vi "FindStartEndPointsRRTImproved.vi"(5 "Robot in":T1, 6 "enemy_robots":T1[](array[typedef]), 7 "ball":dbl[](array[numeric]), 8 "our_robots":T1[](array[typedef]), 9 "Goal":dbl[](array[numeric]), 10 "Initial State":dbl[](array[numeric]), 11 "Collision Points":dbl[][](array[numeric])) -> (2 "Start End Points RRT":dbl[][](array[numeric]))   [LabVIEW 2017]
uses:
  Core/AI Robot.ctl
  Intel/Functions Enum.ctl
  Intel/AttackerStates.ctl
  PathDests.ctl
  PathDest.ctl
  <vilib>/Analysis/_algsub.llb/Real Vector Norm.vi
  <vilib>/Analysis/NI_AALPro.lvlib
panel:
  in  "tamanho minimo":dbl=300.0 format="%#_13g"
  in  "threshold":dbl=50.0 format="%#_13g"
  out "Collision Points \nordenado":dbl[][](array[numeric])
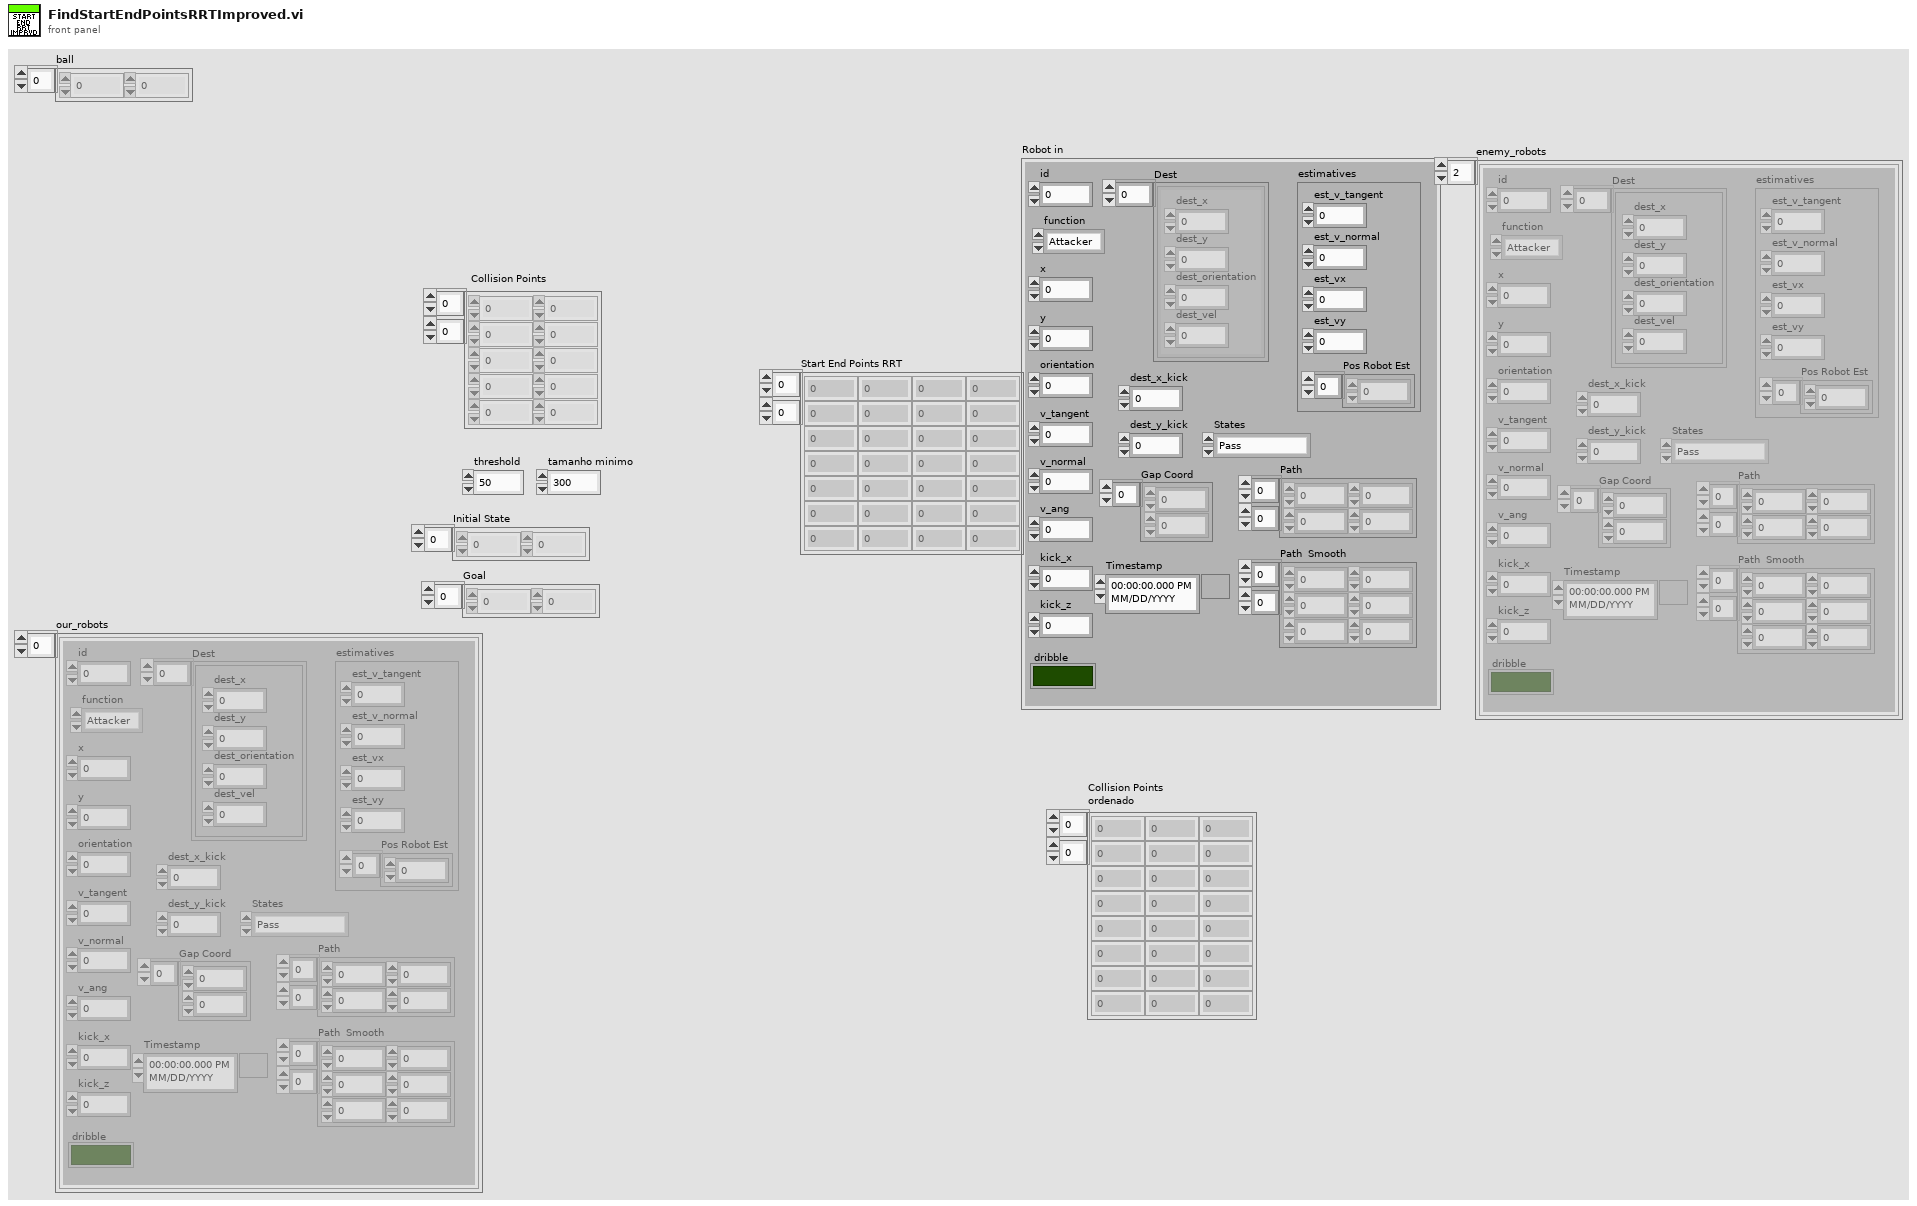
[diagram p1: front panel]
types:
  T1 = typedef "AI Robot.ctl" = cluster{"id":u32, "function":T2, "x":dbl, "y":dbl, "orientation":dbl, "v_tangent":dbl, "v_normal":dbl, "v_ang":dbl, "kick_x":dbl, "kick_z":dbl, "dribble":bool, "Timestamp":timestamp, "estimatives":cluster{"est_v_tangent":dbl, "est_v_normal":dbl, "est_vx":dbl, "est_vy":dbl, "Pos Robot Est":dbl[]}, "dest_x_kick":dbl, "dest_y_kick":dbl, "Gap Coord":dbl[], "States":T3, "Path ":dbl[][], "Path  Smooth":dbl[][], "Dest":T4}
  T2 = typedef "Functions Enum.ctl" = enum16{"Attacker", "Goalie", "Defender", "Striker", "Goto 0", "Dummy", "Kicker", "ZigZag 0", "ZigZag 1", "ZigZag 2", "ZigZag 3", "ZigZag 4", "ZigZag 5", "ZigZag 6", "ZigZag 7", "ZigZag 8", ""}
  T3 = typedef "AttackerStates.ctl" = enum16{"Pass", "GoToTangent", "BallGetting", "GoToKick", ""}
  T4 = typedef "PathDests.ctl" = T5[]
  T5 = typedef "PathDest.ctl" = cluster{"dest_x":dbl, "dest_y":dbl, "dest_orientation":dbl, "dest_vel":dbl}
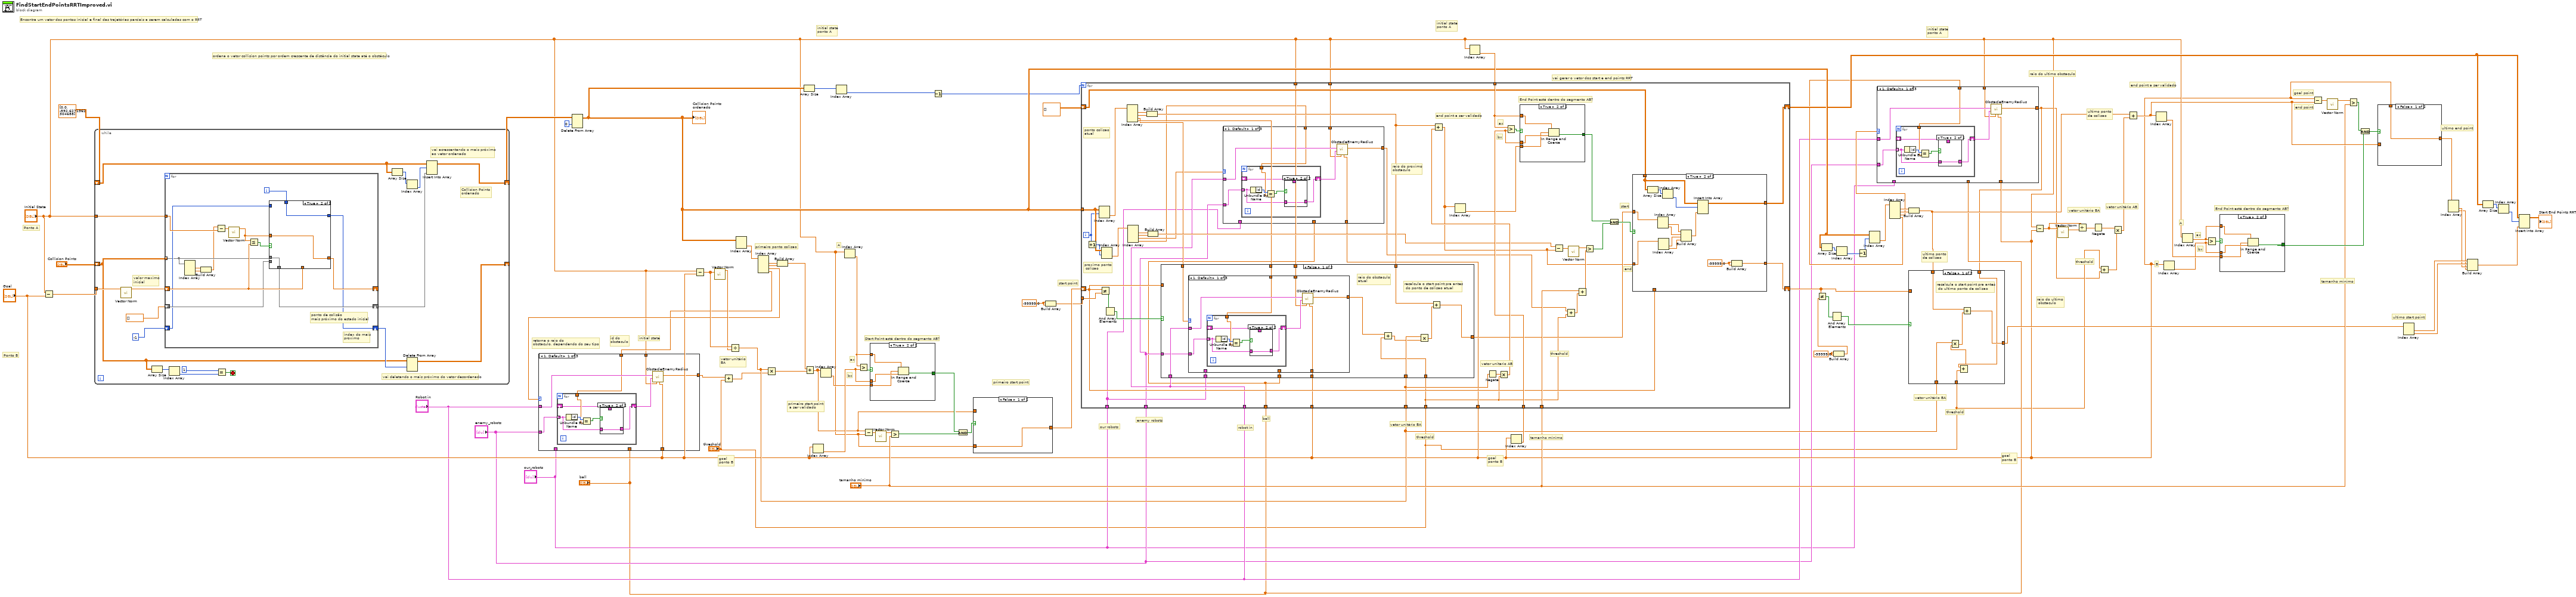
[diagram p0: block diagram]
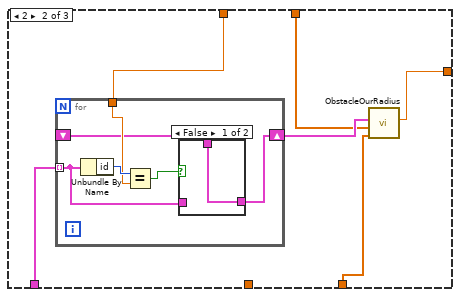
[diagram p3: hidden frame]
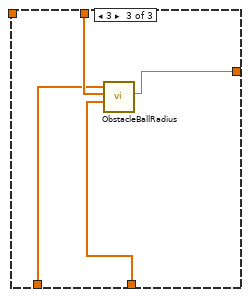
[diagram p5: hidden frame]
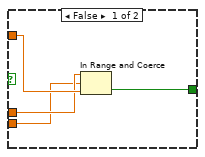
[diagram p6: hidden frame]
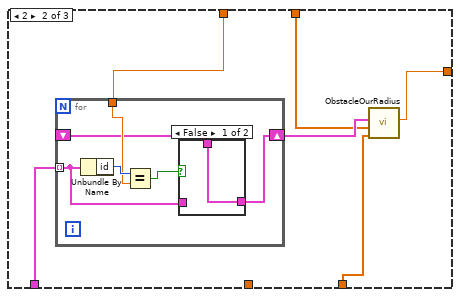
[diagram p10: hidden frame]
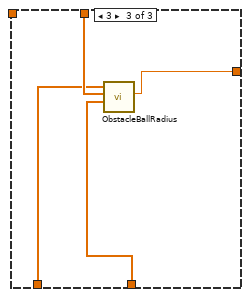
[diagram p12: hidden frame]
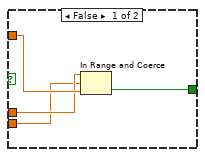
[diagram p14: hidden frame]
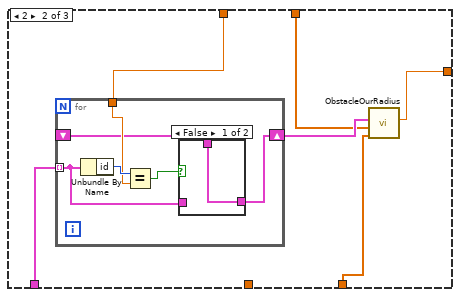
[diagram p16: hidden frame]
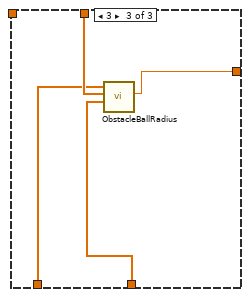
[diagram p18: hidden frame]
diagram:
  w46 = -99999.0 ("element")
  w51 = -99999.0 ("element")
  # "raio do ultimo\n obstaculo"
  # "raio do ultimo obstaculo"
  # "ball"
  # "robot in"
  # "enemy robots"
  # "our robots"
  # "initial state"
  # "id do\nobstaculo"
  # "retorna o raio do \nobstaculo, dependendo do seu tipo"
  # "vai gerar o vetor dos start e end points RRT"
  # "ultimo start point"
  # "ultimo end point"
  # "tamanho minimo"
  # "end point a ser validado"
  # "ultimo ponto\nde colisao"
  # "threshold"
  # "goal\nponto B"
  # "initial state\nponto A"
  # "ultimo ponto\nde colisao"
  # "threshold"
  # "vetor unitário BA"
  # "tamanho minimo"
  # "initial state\nponto A"
  # "goal\nponto B"
  # "threshold"
  # "vetor unitário BA"
  # "start point"
  # "primeiro start point"
  # "A"
  # "Start Point está dentro do segmento AB?"
  # "bx"
  # "ax"
  # "primeiro start point\n a ser validado"
  # "primeiro ponto colisao"
  # "vetor unitário\nBA"
  # "initial state\nponto A"
  # "goal\nponto B"
  # "ordena o vetor collision points por ordem crescente de distância do initial state até o obstáculo"
  # "Encontra um vetor dos pontos inicial e final das trajetórias parciais a serem calculadas com o RRT"
  # "end point"
  # "goal point"
  # "End Point está dentro do segmento AB?"
  # "bx"
  # "ax"
  # "B"
  # "A"
  # "vetor unitário AB"
  # "vetor unitário BA"
  # "Ponto B"
  # "Ponto A"
  n1 = Subtract(x="Initial State", y="Goal") -> (x-y=w87:dbl[])
  n2 = while {
    tunnel: w87 -> [w104]
    tunnel: "Initial State" -> [w101]
    shift-right: [w97] -> w68
    shift-left: dbl[][] [[0.0, -592.6271362304688]] ("Collision Points") -> [w99]
    shift-right: [w93] -> _
    shift-left: "Collision Points" -> [w92]
    stop <- w89 stop-if-true
    # "vai acrescentando o mais próximo\nao vetor ordenado"
    # "vai deletando o mais próximo do vetor desordenado"
    # "Collision Points \nordenado"
    # "valor maximo\ninicial"
    n3 = call-poly <vilib>:"Vector Norm.vi"("Input Vector"=w104) -> ("norm"=w103:dbl)  [unwired: 9 in, 1 out]
    n4 = Array Size(array=w92) -> (size(s)=w91:i32[])
    n5 = for {
      tunnel: w92 -> [w108] mode=indexing
      tunnel: w101 -> [w112]
      shift-right: [w116] -> _
      shift-left: w103 -> [w117]
      shift-right: [w115] -> w98
      shift-left: dbl[] [] ("Goal 2") -> [w114]
      shift-right: [w110] -> w94
      shift-left: -1 -> [w109]
      i -> [w111]
      # "index do mais\nproximo"
      # "ponto de colisão \nmais próximo do estado inicial"
      n6 = Index Array(array=w108) -> (element #1=w107:dbl, element #2=w106:dbl)  [unwired: 3 in, 1 out]
      n7 = Build Array(w107, w106) -> (w105:dbl[])
      n8 = Subtract(x=w105, y=w112) -> (x-y=w119:dbl[])
      n9 = call-poly <vilib>:"Vector Norm.vi"("Input Vector"=w119) -> ("norm"=w113:dbl)  [unwired: 9 in, 1 out]
      n10 = Less Or Equal?(x=w113, y=w117) -> (x <= y?=w118:bool)
      n11 = case shown="True" w118 {
        tunnel: [w122 w125] -> w116
        tunnel: w113 -> [_ w125]
        tunnel: w117 -> [w122 _]
        tunnel: w108 -> [_ w124]
        tunnel: [w121 w124] -> w115
        tunnel: w114 -> [w121 _]
        tunnel: w111 -> [_ w123]
        tunnel: [w120 w123] -> w110
        tunnel: w109 -> [w120 _]
        frame False {
        }
        frame True {
        }
      }
    }
    n12 = Index Array(array=w91) -> (element=w90:i32)  [unwired: 1 in]
    n13 = Equal?(x=1, y=w90) -> (x = y?=w89:bool)
    n14 = Array Size(array=w99) -> (size(s)=w96:i32[])
    n15 = Index Array(array=w96) -> (element=w95:i32)  [unwired: 1 in]
    n16 = Delete From Array(array=w92, index (row)=w94) -> (array with subset deleted=w93:dbl[][])  [unwired: 2 in, 1 out]
    n17 = Insert Into Array(array=w99, index (row)=w95, new element=w98) -> (w97:dbl[][])  [unwired: 1 in]
  }
  n18 = Delete From Array(array=w68, index (row)=0) -> (array with subset deleted=w41:dbl[][])  [unwired: 2 in, 1 out]
  "Collision Points \nordenado" <- w41
  n19 = Subtract(x="Initial State", y="Goal") -> (x-y=w65:dbl[])
  n20 = call-poly <vilib>:"Vector Norm.vi"("Input Vector"=w65) -> ("norm"=w64:dbl)  [unwired: 9 in, 1 out]
  n21 = Divide(x=w65, y=w64) -> (x/y=w47:dbl[])
  n22 = Index Array(array=w41) -> (element=w21:dbl[])  [unwired: 2 in]
  n23 = Index Array(array=w21) -> (element #1=w23:dbl, element #2=w22:dbl, element #3=w19:dbl, element #4=w18:dbl)  [unwired: 4 in]
  n24 = case shown="1, Default" w19 {
    tunnel: "Robot in" -> [w132 _ _]
    tunnel: "enemy_robots" -> [w131 _ _]
    tunnel: w18 -> [w130 w145 _]
    tunnel: "Goal" -> [w128 w142 w157]
    tunnel: "Initial State" -> [w127 w143 w158]
    tunnel: [w126 w141 w156] -> w16
    tunnel: "our_robots" -> [_ w146 _]
    tunnel: "ball" -> [_ _ w155]
    frame 1, Default {
      n25 = for {
        tunnel: w131 -> [w135] mode=indexing
        shift-right: [w134] -> w129
        shift-left: _ -> [w133]
        tunnel: w130 -> [w137]
        n26 = Unbundle By Name(w135) -> ("id"=w138:u32)
        n27 = Equal?(x=w138, y=w137) -> (x = y?=w136:bool)
        n28 = case shown="True" w136 {
          tunnel: w135 -> [_ w140]
          tunnel: [w139 w140] -> w134
          tunnel: w133 -> [w139 _]
          frame False {
          }
          frame True {
          }
        }
      }
      n29 = call "ObstacleEnemyRadius.vi"("Goal"=w128, "Initial State"=w127, "Robot enemy"=w129, "Robot in"=w132) -> ("obstacle enemy radius"=w126:dbl)  [unwired: 7 in]
    }
    frame 2 {
      n30 = for {
        tunnel: w146 -> [w149] mode=indexing
        shift-right: [w148] -> w144
        shift-left: _ -> [w147]
        tunnel: w145 -> [w151]
        n31 = Unbundle By Name(w149) -> ("id"=w152:u32)
        n32 = Equal?(x=w152, y=w151) -> (x = y?=w150:bool)
        n33 = case shown="False" w150 {
          tunnel: w149 -> [_ w154]
          tunnel: [w153 w154] -> w148
          tunnel: w147 -> [w153 _]
          frame False {
          }
          frame True {
          }
        }
      }
      n34 = call "ObstacleOurRadius.vi"("Goal"=w142, "Initial State"=w143, "other robot"=w144) -> ("obstacle enemy radius"=w141:dbl)  [unwired: 8 in]
    }
    frame 3 {
      n35 = call "ObstacleBallRadius.vi"("Goal"=w157, "Initial State"=w158, "ball"=w155) -> ("obstacle enemy radius"=w156:dbl)  [unwired: 8 in]
    }
  }
  n36 = Add(x=w16, y="threshold") -> (x+y=w17:dbl)
  n37 = Multiply(x=w47, y=w17) -> (x*y=w63:dbl[])
  n38 = Build Array(w23, w22) -> (w20:dbl[])
  n39 = Array Size(array=w41) -> (size(s)=w67:i32[])
  n40 = Add(x=w20, y=w63) -> (x+y=w53:dbl[])
  n41 = Index Array(array="Goal") -> (element=w60:dbl)  [unwired: 1 in]
  n42 = Index Array(array=w53) -> (element=w59:dbl)  [unwired: 1 in]
  n43 = Index Array(array=w67) -> (element=w66:i32)  [unwired: 1 in]
  n44 = Index Array(array="Initial State") -> (element=w61:dbl)  [unwired: 1 in]
  n45 = Greater?(x=w61, y=w60) -> (0:w62:bool)
  n46 = Subtract(x=w53, y="Initial State") -> (x-y=w58:dbl[])
  n47 = case shown="True" w62 {
    tunnel: w61 -> [w162 w166]
    tunnel: w60 -> [w161 w165]
    tunnel: w59 -> [w160 w164]
    tunnel: [w159 w163] -> w56
    frame False {
      n48 = In Range and Coerce(upper limit=w161, x=w160, lower limit=w162) -> (In Range?=w159:bool)  [unwired: 1 out]
    }
    frame True {
      n49 = In Range and Coerce(upper limit=w166, x=w164, lower limit=w165) -> (In Range?=w163:bool)  [unwired: 1 out]
    }
  }
  n50 = call-poly <vilib>:"Vector Norm.vi"("Input Vector"=w58) -> ("norm"=w57:dbl)  [unwired: 9 in, 1 out]
  n51 = Greater?(x=w57, y="tamanho minimo") -> (0:w55:bool)
  n52 = Decrement(x=w66) -> (x-1=w26:i32)
  n53 = And(x=w56, y=w55) -> (x .and. y?=w54:bool)
  n54 = case shown="False" w54 {
    tunnel: [w167 w168] -> w52
    tunnel: w53 -> [_ w168]
    tunnel: "Initial State" -> [w167 _]
    frame False {
    }
    frame True {
    }
  }
  n55 = Build Array(w51, w51) -> (w50:dbl[])
  n56 = Index Array(array="Initial State") -> (element=w49:dbl)  [unwired: 1 in]
  n57 = Index Array(array="Goal") -> (element=w48:dbl)  [unwired: 1 in]
  n58 = for {
    N: w26 -> [_]
    tunnel: w41 -> [w217]
    shift-right: [w195] -> w24
    shift-left: dbl[][] [] -> [w198]
    shift-right: [w194] -> w42
    shift-left: w52 -> [w192]
    tunnel: w50 -> [w214]
    tunnel: w47 -> [w212]
    tunnel: "threshold" -> [w171]
    tunnel: w49 -> [w208]
    tunnel: w48 -> [w207]
    tunnel: "tamanho minimo" -> [w204]
    tunnel: "Initial State" -> [w182]
    tunnel: "our_robots" -> [w173]
    tunnel: "enemy_robots" -> [w176]
    tunnel: "Robot in" -> [w177]
    tunnel: "Goal" -> [w180]
    tunnel: "ball" -> [w172]
    tunnel: "Initial State" -> [w179]
    tunnel: "Goal" -> [w178]
    i -> [w216]
    # "raio do proximo\nobstaculo"
    # "end"
    # "start"
    # "threshold"
    # "End Point está dentro do segmento AB?"
    # "bx"
    # "ax"
    # "end point a ser validado"
    # "vetor unitario AB"
    # "proximo ponto\n colisao"
    # "ponto colisao\natual"
    n59 = Increment(x=w216) -> (x+1=w215:i32)
    n60 = Index Array(array=w217, index (row)=w216) -> (element=w189:dbl[])  [unwired: 1 in]
    n61 = Not Equal?(x=w192, y=w214) -> (x != y?=w213:bool[])
    n62 = Index Array(array=w217, index (row)=w215) -> (element=w185:dbl[])  [unwired: 1 in]
    n63 = And Array Elements(Boolean array=w213) -> (logical AND=w193:bool)
    n64 = Index Array(array=w189) -> (element #1=w191:dbl, element #2=w190:dbl, element #3=w181:dbl, element #4=w183:dbl)  [unwired: 4 in]
    n65 = Index Array(array=w185) -> (element #1=w186:dbl, element #2=w187:dbl, element #3=w175:dbl, element #4=w174:dbl)  [unwired: 4 in]
    n66 = Build Array(w191, w190) -> (w188:dbl[])
    n67 = Build Array(w186, w187) -> (w184:dbl[])
    n68 = case shown="False" w193 {
      tunnel: w192 -> [_ w322]
      tunnel: [w285 w322] -> w197
      tunnel: w212 -> [w288 _]
      tunnel: w171 -> [w281 _]
      tunnel: w188 -> [w287 _]
      tunnel: w183 -> [w284 _]
      tunnel: w182 -> [w283 _]
      tunnel: w181 -> [w279 _]
      tunnel: w177 -> [w278 _]
      tunnel: w176 -> [w277 _]
      tunnel: w180 -> [w276 _]
      tunnel: w173 -> [w275 _]
      tunnel: w172 -> [w274 _]
      frame False {
        # "raio do obstaculo\natual"
        # "recalcula o start point pra antes\n do ponto de colisao atual"
        n69 = case shown="1, Default" w279 {
          tunnel: w278 -> [w295 _ _]
          tunnel: w277 -> [w294 _ _]
          tunnel: w284 -> [w293 w308 _]
          tunnel: w276 -> [w291 w305 w320]
          tunnel: w283 -> [w290 w306 w321]
          tunnel: [w289 w304 w319] -> w282
          tunnel: w275 -> [_ w309 _]
          tunnel: w274 -> [_ _ w318]
          frame 1, Default {
            n70 = for {
              tunnel: w294 -> [w298] mode=indexing
              shift-right: [w297] -> w292
              shift-left: _ -> [w296]
              tunnel: w293 -> [w300]
              n71 = Unbundle By Name(w298) -> ("id"=w301:u32)
              n72 = Equal?(x=w301, y=w300) -> (x = y?=w299:bool)
              n73 = case shown="True" w299 {
                tunnel: w298 -> [_ w303]
                tunnel: [w302 w303] -> w297
                tunnel: w296 -> [w302 _]
                frame False {
                }
                frame True {
                }
              }
            }
            n74 = call "ObstacleEnemyRadius.vi"("Goal"=w291, "Initial State"=w290, "Robot enemy"=w292, "Robot in"=w295) -> ("obstacle enemy radius"=w289:dbl)  [unwired: 7 in]
          }
          frame 2 {
            n75 = for {
              tunnel: w309 -> [w312] mode=indexing
              shift-right: [w311] -> w307
              shift-left: _ -> [w310]
              tunnel: w308 -> [w314]
              n76 = Unbundle By Name(w312) -> ("id"=w315:u32)
              n77 = Equal?(x=w315, y=w314) -> (x = y?=w313:bool)
              n78 = case shown="False" w313 {
                tunnel: w312 -> [_ w317]
                tunnel: [w316 w317] -> w311
                tunnel: w310 -> [w316 _]
                frame False {
                }
                frame True {
                }
              }
            }
            n79 = call "ObstacleOurRadius.vi"("Goal"=w305, "Initial State"=w306, "other robot"=w307) -> ("obstacle enemy radius"=w304:dbl)  [unwired: 8 in]
          }
          frame 3 {
            n80 = call "ObstacleBallRadius.vi"("Goal"=w320, "Initial State"=w321, "ball"=w318) -> ("obstacle enemy radius"=w319:dbl)  [unwired: 8 in]
          }
        }
        n81 = Add(x=w282, y=w281) -> (x+y=w280:dbl)
        n82 = Multiply(x=w288, y=w280) -> (x*y=w286:dbl[])
        n83 = Add(x=w287, y=w286) -> (x+y=w285:dbl[])
      }
      frame True {
        # "start  point ainda é valido, \ne nao precisa recalcular"
      }
    }
    n84 = case shown="1, Default" w175 {
      tunnel: w177 -> [w224 _ _]
      tunnel: w176 -> [w223 _ _]
      tunnel: w174 -> [w222 w237 _]
      tunnel: w178 -> [w220 w234 w249]
      tunnel: w179 -> [w219 w235 w250]
      tunnel: [w218 w233 w248] -> w170
      tunnel: w173 -> [_ w238 _]
      tunnel: w172 -> [_ _ w247]
      frame 1, Default {
        n85 = for {
          tunnel: w223 -> [w227] mode=indexing
          shift-right: [w226] -> w221
          shift-left: _ -> [w225]
          tunnel: w222 -> [w229]
          n86 = Unbundle By Name(w227) -> ("id"=w230:u32)
          n87 = Equal?(x=w230, y=w229) -> (x = y?=w228:bool)
          n88 = case shown="True" w228 {
            tunnel: w227 -> [_ w232]
            tunnel: [w231 w232] -> w226
            tunnel: w225 -> [w231 _]
            frame False {
            }
            frame True {
            }
          }
        }
        n89 = call "ObstacleEnemyRadius.vi"("Goal"=w220, "Initial State"=w219, "Robot enemy"=w221, "Robot in"=w224) -> ("obstacle enemy radius"=w218:dbl)  [unwired: 7 in]
      }
      frame 2 {
        n90 = for {
          tunnel: w238 -> [w241] mode=indexing
          shift-right: [w240] -> w236
          shift-left: _ -> [w239]
          tunnel: w237 -> [w243]
          n91 = Unbundle By Name(w241) -> ("id"=w244:u32)
          n92 = Equal?(x=w244, y=w243) -> (x = y?=w242:bool)
          n93 = case shown="False" w242 {
            tunnel: w241 -> [_ w246]
            tunnel: [w245 w246] -> w240
            tunnel: w239 -> [w245 _]
            frame False {
            }
            frame True {
            }
          }
        }
        n94 = call "ObstacleOurRadius.vi"("Goal"=w234, "Initial State"=w235, "other robot"=w236) -> ("obstacle enemy radius"=w233:dbl)  [unwired: 8 in]
      }
      frame 3 {
        n95 = call "ObstacleBallRadius.vi"("Goal"=w249, "Initial State"=w250, "ball"=w247) -> ("obstacle enemy radius"=w248:dbl)  [unwired: 8 in]
      }
    }
    n96 = Negate(x=w212) -> (-x=w211:dbl[])
    n97 = Multiply(x=w211, y=w171) -> (x*y=w210:dbl[])
    n98 = Add(x=w188, y=w210) -> (x+y=w196:dbl[])
    n99 = Index Array(array=w196) -> (element=w200:dbl)  [unwired: 1 in]
    n100 = Greater?(x=w208, y=w207) -> (0:w209:bool)
    n101 = case shown="True" w209 {
      tunnel: w208 -> [w269 w273]
      tunnel: w207 -> [w268 w272]
      tunnel: w200 -> [w267 w271]
      tunnel: [w266 w270] -> w202
      frame False {
        n102 = In Range and Coerce(upper limit=w268, x=w267, lower limit=w269) -> (In Range?=w266:bool)  [unwired: 1 out]
      }
      frame True {
        n103 = In Range and Coerce(upper limit=w273, x=w271, lower limit=w272) -> (In Range?=w270:bool)  [unwired: 1 out]
      }
    }
    n104 = Subtract(x=w184, y=w196) -> (x-y=w206:dbl[])
    n105 = Add(x=w170, y=w171) -> (x+y=w169:dbl)
    n106 = call-poly <vilib>:"Vector Norm.vi"("Input Vector"=w206) -> ("norm"=w205:dbl)  [unwired: 9 in, 1 out]
    n107 = Add(x=w204, y=w169) -> (x+y=w203:dbl)
    n108 = Greater?(x=w205, y=w203) -> (0:w201:bool)
    n109 = And(x=w202, y=w201) -> (x .and. y?=w199:bool)
    n110 = case shown="True" w199 {
      tunnel: w198 -> [w252 w264]
      tunnel: w197 -> [_ w262]
      tunnel: w196 -> [_ w261]
      tunnel: [w252 w255] -> w195
      tunnel: [w251 w253] -> w194
      tunnel: w192 -> [w251 _]
      frame False {
      }
      frame True {
        w254 = -99999.0 ("element")
        n111 = Array Size(array=w264) -> (size(s)=w265:i32[])
        n112 = Index Array(array=w262) -> (element #1=w260:dbl, element #2=w259:dbl)  [unwired: 2 in]
        n113 = Index Array(array=w261) -> (element #1=w258:dbl, element #2=w257:dbl)  [unwired: 2 in]
        n114 = Index Array(array=w265) -> (element=w263:i32)  [unwired: 1 in]
        n115 = Build Array(w260, w259, w258, w257) -> (w256:dbl[])
        n116 = Insert Into Array(array=w264, index (row)=w263, new element=w256) -> (w255:dbl[][])  [unwired: 1 in]
        n117 = Build Array(w254, w254) -> (w253:dbl[])
      }
    }
  }
  n118 = Array Size(array=w41) -> (size(s)=w40:i32[])
  n119 = Build Array(w46, w46) -> (w45:dbl[])
  n120 = Not Equal?(x=w42, y=w45) -> (x != y?=w44:bool[])
  n121 = And Array Elements(Boolean array=w44) -> (logical AND=w43:bool)
  n122 = Index Array(array=w40) -> (element=w39:i32)  [unwired: 1 in]
  n123 = Decrement(x=w39) -> (x-1=w38:i32)
  n124 = Index Array(array=w41, index (row)=w38) -> (element=w13:dbl[])  [unwired: 1 in]
  n125 = Index Array(array=w13) -> (element #1=w15:dbl, element #2=w14:dbl, element #3=w11:dbl, element #4=w10:dbl)  [unwired: 4 in]
  n126 = case shown="1, Default" w11 {
    tunnel: "Robot in" -> [w329 _ _]
    tunnel: "enemy_robots" -> [w328 _ _]
    tunnel: w10 -> [w327 w342 _]
    tunnel: "Goal" -> [w325 w339 w354]
    tunnel: "Initial State" -> [w324 w340 w355]
    tunnel: [w323 w338 w353] -> w1
    tunnel: "our_robots" -> [_ w343 _]
    tunnel: "ball" -> [_ _ w352]
    frame 1, Default {
      n127 = for {
        tunnel: w328 -> [w332] mode=indexing
        shift-right: [w331] -> w326
        shift-left: _ -> [w330]
        tunnel: w327 -> [w334]
        n128 = Unbundle By Name(w332) -> ("id"=w335:u32)
        n129 = Equal?(x=w335, y=w334) -> (x = y?=w333:bool)
        n130 = case shown="True" w333 {
          tunnel: w332 -> [_ w337]
          tunnel: [w336 w337] -> w331
          tunnel: w330 -> [w336 _]
          frame False {
          }
          frame True {
          }
        }
      }
      n131 = call "ObstacleEnemyRadius.vi"("Goal"=w325, "Initial State"=w324, "Robot enemy"=w326, "Robot in"=w329) -> ("obstacle enemy radius"=w323:dbl)  [unwired: 7 in]
    }
    frame 2 {
      n132 = for {
        tunnel: w343 -> [w346] mode=indexing
        shift-right: [w345] -> w341
        shift-left: _ -> [w344]
        tunnel: w342 -> [w348]
        n133 = Unbundle By Name(w346) -> ("id"=w349:u32)
        n134 = Equal?(x=w349, y=w348) -> (x = y?=w347:bool)
        n135 = case shown="False" w347 {
          tunnel: w346 -> [_ w351]
          tunnel: [w350 w351] -> w345
          tunnel: w344 -> [w350 _]
          frame False {
          }
          frame True {
          }
        }
      }
      n136 = call "ObstacleOurRadius.vi"("Goal"=w339, "Initial State"=w340, "other robot"=w341) -> ("obstacle enemy radius"=w338:dbl)  [unwired: 8 in]
    }
    frame 3 {
      n137 = call "ObstacleBallRadius.vi"("Goal"=w354, "Initial State"=w355, "ball"=w352) -> ("obstacle enemy radius"=w353:dbl)  [unwired: 8 in]
    }
  }
  n138 = Build Array(w15, w14) -> (w12:dbl[])
  n139 = case shown="False" w43 {
    tunnel: w42 -> [_ w363]
    tunnel: [w360 w363] -> w35
    tunnel: w47 -> [w362 _]
    tunnel: "threshold" -> [w358 _]
    tunnel: w12 -> [w359 _]
    tunnel: w1 -> [w357 _]
    frame False {
      # "recalcula o start point pra antes\n do ultimo ponto de colisao"
      n140 = Add(x=w357, y=w358) -> (x+y=w356:dbl)
      n141 = Multiply(x=w362, y=w356) -> (x*y=w361:dbl[])
      n142 = Add(x=w359, y=w361) -> (x+y=w360:dbl[])
    }
    frame True {
      # "start  point ainda é valido, \ne nao precisa recalcular"
    }
  }
  n143 = Subtract(x="Initial State", y="Goal") -> (x-y=w86:dbl[])
  n144 = call-poly <vilib>:"Vector Norm.vi"("Input Vector"=w86) -> ("norm"=w85:dbl)  [unwired: 9 in, 1 out]
  n145 = Divide(x=w86, y=w85) -> (x/y=w82:dbl[])
  n146 = Negate(x=w82) -> (-x=w84:dbl[])
  n147 = Add(x="threshold", y=w1) -> (x+y=w2:dbl)
  n148 = Multiply(x=w84, y=w2) -> (x*y=w83:dbl[])
  n149 = Add(x=w12, y=w83) -> (x+y=w72:dbl[])
  n150 = Index Array(array=w72) -> (element=w81:dbl)  [unwired: 1 in]
  n151 = Index Array(array="Goal") -> (element=w79:dbl)  [unwired: 1 in]
  n152 = Index Array(array="Initial State") -> (element=w78:dbl)  [unwired: 1 in]
  n153 = Greater?(x=w78, y=w79) -> (0:w80:bool)
  n154 = case shown="True" w80 {
    tunnel: w78 -> [w367 w371]
    tunnel: w79 -> [w366 w370]
    tunnel: w81 -> [w365 w369]
    tunnel: [w364 w368] -> w75
    frame False {
      n155 = In Range and Coerce(upper limit=w366, x=w365, lower limit=w367) -> (In Range?=w364:bool)  [unwired: 1 out]
    }
    frame True {
      n156 = In Range and Coerce(upper limit=w371, x=w369, lower limit=w370) -> (In Range?=w368:bool)  [unwired: 1 out]
    }
  }
  n157 = Subtract(x="Goal", y=w72) -> (x-y=w77:dbl[])
  n158 = call-poly <vilib>:"Vector Norm.vi"("Input Vector"=w77) -> ("norm"=w76:dbl)  [unwired: 9 in, 1 out]
  n159 = Greater?(x=w76, y="tamanho minimo") -> (0:w74:bool)
  n160 = And(x=w74, y=w75) -> (x .and. y?=w73:bool)
  n161 = case shown="False" w73 {
    tunnel: w72 -> [_ w373]
    tunnel: [w372 w373] -> w36
    tunnel: "Goal" -> [w372 _]
    frame False {
    }
    frame True {
    }
  }
  n162 = Index Array(array=w35) -> (element #1=w34:dbl, element #2=w33:dbl)  [unwired: 2 in]
  n163 = Index Array(array=w36) -> (element #1=w32:dbl, element #2=w31:dbl)  [unwired: 2 in]
  n164 = Build Array(w34, w33, w32, w31) -> (w28:dbl[])
  n165 = Array Size(array=w24) -> (size(s)=w30:i32[])
  n166 = Index Array(array=w30) -> (element=w29:i32)  [unwired: 1 in]
  n167 = Insert Into Array(array=w24, index (row)=w29, new element=w28) -> (→"Start End Points RRT":dbl[][])  [unwired: 1 in]
